vi "LoadFileCore.vi"(8 "error in (no error)":errorcluster, 10 "ErrorUX CSV File Path":path, 11 "LabErrorUX in":refnum<class "LabErrorUX.lvclass">) -> (0 "error out":errorcluster, 3 "LabErrorUX out":refnum<class "LabErrorUX.lvclass">)   [LabVIEW 2019, in "LabErrorUX.lvclass"]
uses:
  LabErrorUX.lvclass
  <vilib>/SLL Toolkit/SLL File IO/Spreadsheet/SLL Spreadsheet.lvlib
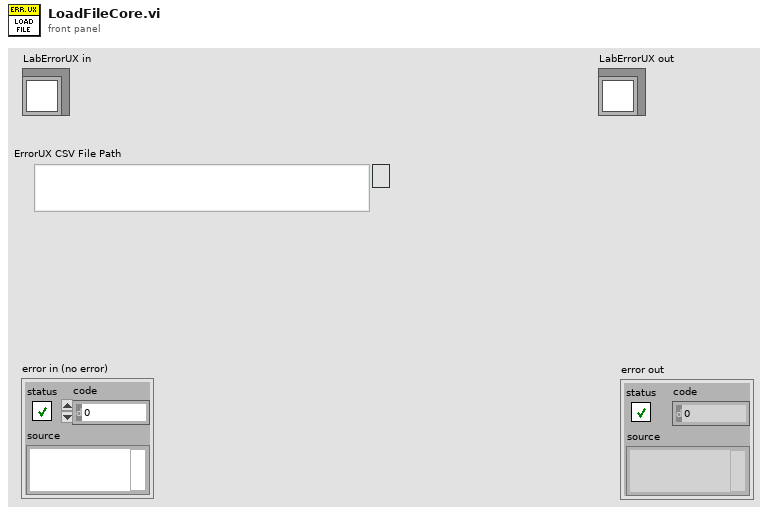
[diagram p1: front panel]
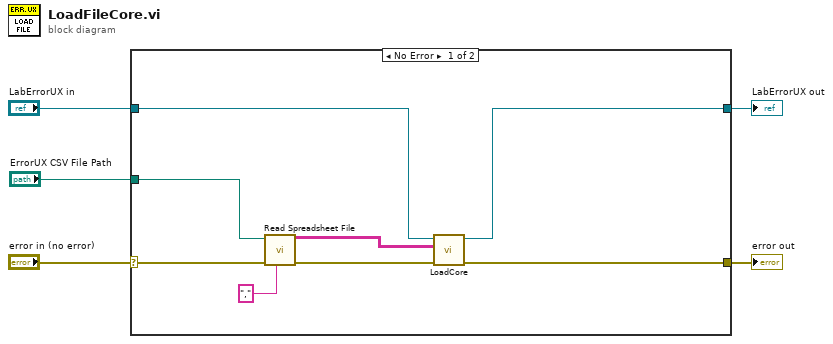
[diagram p0: block diagram]
diagram:
  n1 = case shown="No Error" "error in (no error)" {
    selector: "error in (no error)" -> [w9 w15]
    tunnel: [w13 w15] -> w4
    tunnel: [w11 w14] -> w2
    tunnel: "LabErrorUX in" -> [w12 w14]
    tunnel: "ErrorUX CSV File Path" -> [w8 _]
    frame No Error {
      n2 = call <vilib>:"Read Spreadsheet File.vi"("Delimiter (tab)"=",", "error in (no error)"=w9, "File Path"=w8) -> ("error out"=w10:errorcluster, "2D Array"=w7:string[][])  [unwired: 7 in]
      n3 = call-dynamic "LoadCore.vi"("error in (no error)"=w10, "ErrorDetails"=w7, "LabErrorUX in"=w12) -> ("error out"=w13:errorcluster, "LabErrorUX out"=w11:refnum<class "LabErrorUX.lvclass">)  [unwired: 7 in]
    }
    frame Error {
    }
  }
  "error out" <- w4
  "LabErrorUX out" <- w2
